vi "OAT Tachless Get Default Refine Bandwidth.vi"(8 "min RPM":dbl format="%.2f", 9 "Window Length":T2(ring)=enum."512", 10 "Default Mask \nWidth (Pixels)":i32=3, 11 "Sample Rate (Hz)":dbl) -> (2 "bandwidth":T1={"bandwidth value"=0.5, "bandwidth unit"=enum."Order"} {"bandwidth value" min=0.0 format="%.2f"})   [LabVIEW 2017, in "SoundVib_Tachless.lvlib"]
uses:
  <vilib>/addons/Sound and Vibration/Order Analysis/Tachless/SoundVib_Tachless.lvlib
  <vilib>/addons/Sound and Vibration/Order Analysis/Ref Gabor Order Tracking/Mask Bandwidth.ctl
  <vilib>/addons/Sound and Vibration/Order Analysis/Gabor Order Tracking/SoundVib_Gabor.lvlib
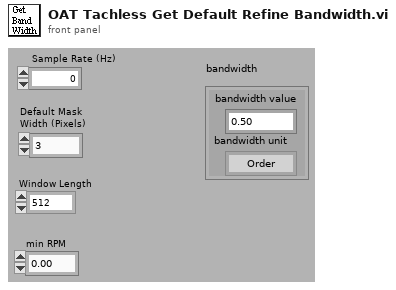
[diagram p1: front panel]
types:
  T1 = typedef "SoundVib_Gabor.lvlib/Mask Bandwidth.ctl" = cluster{"bandwidth value":dbl, "bandwidth unit":enum16{"Order", "Hz"}}
  T2 = enum16{"256", "512", "1024", "2048", "4096", "8192", "16384", "32768"}
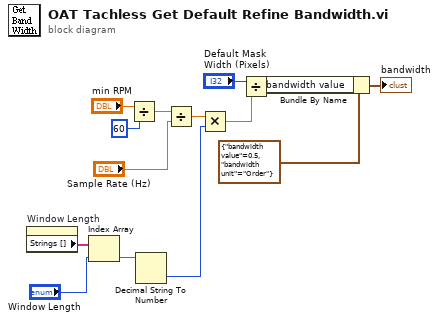
[diagram p0: block diagram]
diagram:
  n1 = property on="Window Length" class="Enum (strict)"() -> ("Strings []"=w9:string[])  [unwired: 2 in, 2 out]
  n2 = Index Array(array=w9, index="Window Length") -> (element=w7:string)
  n3 = Divide(x="min RPM", y=60) -> (x/y=w12:dbl)
  n4 = Decimal String To Number(string=w7) -> (number=w6:i32)  [unwired: 2 in, 1 out]
  n5 = Divide(x=w12, y="Sample Rate (Hz)") -> (x/y=w10:dbl)
  n6 = Multiply(x=w10, y=w6) -> (x*y=w4:dbl)
  n7 = Divide(x="Default Mask \nWidth (Pixels)", y=w4) -> (x/y=w2:dbl)
  n8 = Bundle By Name(cluster=T1 {"bandwidth value"=0.5, "bandwidth unit"=enum."Order"} ("bandwidth"), "bandwidth value"=w2) -> (→"bandwidth":T1)
